vi "GetMetadataValue.vi"(7 "DLL path":path, 8 "error in (no error)":errorcluster, 10 "key":string, 11 "session id in":i32) -> (0 "error out":errorcluster, 1 "MetadataValue":string, 3 "session id out":i32)   [LabVIEW 2017, in "ONNX Class Library.lvlib"]
doc: "/**\n * @brief Получить значение метаданных по ключу\n * \n * @param sessionId [IN] ID сессии\n * @param key [IN] Ключ метаданных (например, \"producer_name\")\n * @param buffer [OUT] Буфер для строки со значением\n * @param bufferSize [IN] Размер буфера (рекомендуется 256)\n * \n * @return int32: 0 при успехе\n * @return int32: -1 если ключ не найден\n */\nint GetMetadataValue(int sessionId, const char* key, char* buffer, int bufferSize);"
uses:
  ONNX Class Library.lvlib
panel:
  out "bufferSize":i32
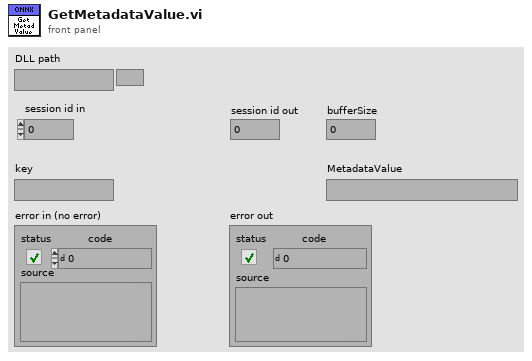
[diagram p1: front panel]
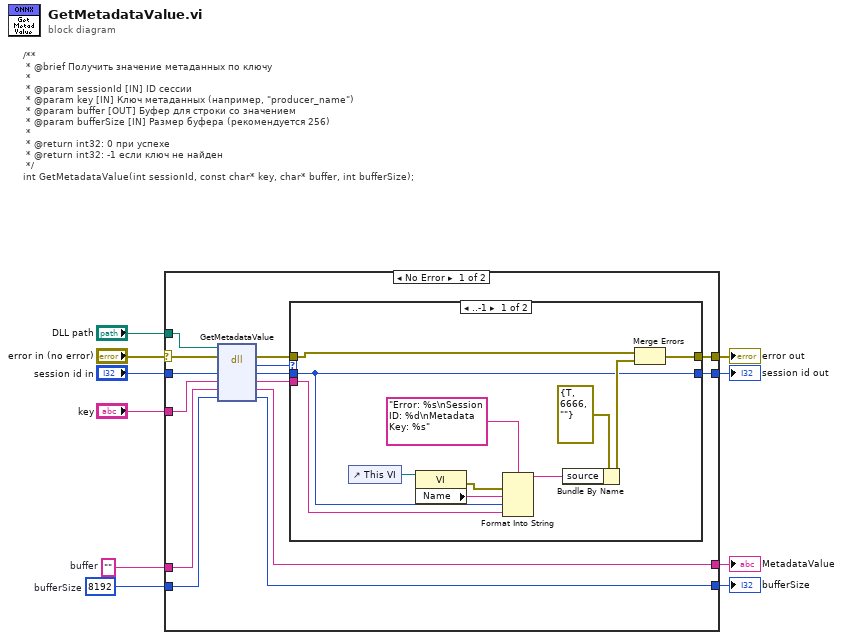
[diagram p0: block diagram]
diagram:
  w7 = 8192  # bufferSize
  w8 = ""  # buffer
  # "/**\n * @brief Получить значение метаданных по ключу\n * \n * @param sessionId [IN] ID сессии\n * @param key [IN] Ключ метаданных (например, \"producer_name\")\n * @param buffer [OUT] Буфер для строки со значением\n * @param bufferSize [IN] Размер буфера (рекомендуется 256)\n * \n * @return int32: 0 при успехе\n * @return int32: -1 если ключ не найден\n */\nint GetMetadataValue(int sessionId, const char* key, char* buffer, int bufferSize);"
  n1 = case shown="No Error" "error in (no error)" {
    selector: "error in (no error)" -> [w11 w39]
    tunnel: "session id in" -> [w24 w38]
    tunnel: "key" -> [w23 _]
    tunnel: w8 -> [w22 _]
    tunnel: w7 -> [w21 _]
    tunnel: [w20 _] -> w6
    tunnel: [w19 _] -> w5
    tunnel: [w17 w39] -> w4
    tunnel: [w16 w38] -> w3
    tunnel: "DLL path" -> [w12 _]
    frame No Error {
      n2 = dll-call lib="home/ivan/LabVIEWData/ONNX/Test/libonnx_wrapper/unix64/libonnx_wrapper.*" fn="GetMetadataValue"(path in=w12, error in=w11, "sessionId"=w24, "key"=w23, "buffer"=w22, "bufferSize"=w21) -> (error out=w18:errorcluster, "return"=w15:i32, "sessionId"=w14:i32, "key"=w13:string, "buffer"=w20:string, "bufferSize"=w19:i32)  [unwired: 1 in, 1 out]
      n3 = case shown="..-1" w15 {
        tunnel: w18 -> [w26 w37]
        tunnel: [w27 w37] -> w17
        tunnel: w14 -> [w28 w36]
        tunnel: [w28 w36] -> w16
        tunnel: w13 -> [w25 _]
        frame ..-1 {
          n4 = control-ref of="This VI"() -> (w32:refnum<vi>)
          n5 = property class="VI"(reference=w32) -> (error out=w29:errorcluster, "Name"=w31:string)  [unwired: 1 in, 1 out]
          n6 = Format Into String(format string="Error: %s\nSession ID: %d\nMetadata Key: %s", error in=w29, w31, w28, w25) -> (resulting string=w33:string)  [unwired: 1 in, 1 out]
          n7 = Bundle By Name(cluster=errorcluster {"status"=TRUE, "code"=6666, "source"=""} ("error out"), "source"=w33) -> (w34:errorcluster)
          n8 = Merge Errors(w26, w34) -> (w27:errorcluster)
        }
        frame 0.. {
        }
      }
    }
    frame Error {
    }
  }
  "error out" <- w4
  "session id out" <- w3
  "MetadataValue" <- w6
  "bufferSize" <- w5
